vi "_031.vi"() -> ()   [LabVIEW 2024]
panel:
  out "Numeric":dbl
  in  "Array":dbl[](array[numeric])
  # "To make last array element size Times 2 :"
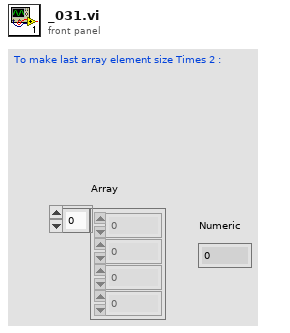
[diagram p1: front panel]
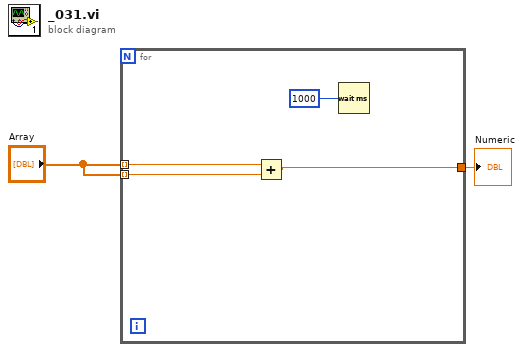
[diagram p0: block diagram]
diagram:
  n1 = for {
    tunnel: "Array" -> [w6] mode=indexing
    tunnel: "Array" -> [w5] mode=indexing
    tunnel: [w4] -> w1
    n2 = Add(x=w6, y=w5) -> (x+y=w4:dbl)
    n3 = Wait (ms)(milliseconds to wait=u32 1000 ("millisecond timer value")) -> ()  [unwired: 1 out]
  }
  "Numeric" <- w1
